vi "Counter 32 Bit (HOST) (SubVI).vi"(5 "Auto RESET":bool=TRUE, 7 "RESET":bool, 8 "Enable":bool, 11 "Max. Count":u32=4294967295) -> (1 "Count End?":bool, 2 "Count Begin?":bool, 3 "Count":u32)   [LabVIEW 2020]
panel:
  # "Counter 32:\n\nCounts when Enable input is TRUE. Count value is 0-indexed."
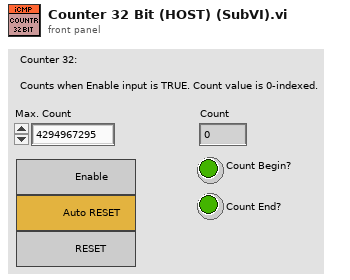
[diagram p1: front panel]
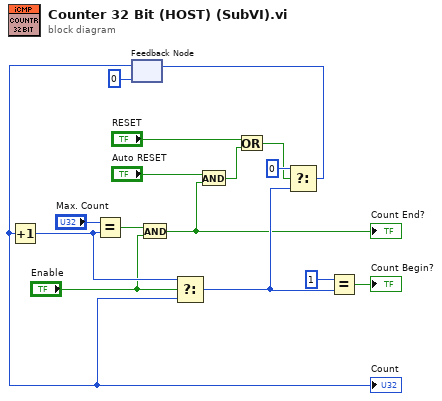
[diagram p0: block diagram]
diagram:
  n1 = feedback #1(u32 0) -> (w16:u32)
  "Count" <- w16
  n2 = Increment(x=w16) -> (x+1=w3:u32)
  n3 = Equal?(x="Max. Count", y=w3) -> (x = y?=w9:bool)
  n4 = And(x=w9, y="Enable") -> (x .and. y?=w2:bool)
  "Count End?" <- w2
  n5 = Select(t=w3, s="Enable", f=w16) -> (s? t:f=w7:u32)
  n6 = And(x="Auto RESET", y=w2) -> (x .and. y?=w5:bool)
  n7 = Or(x="RESET", y=w5) -> (x .or. y?=w4:bool)
  n8 = Select(t=u32 0, s=w4, f=w7) -> (s? t:f=w8:u32)
  n9 = feedback-in #1(w8) -> ()
  n10 = Equal?(x=u32 1, y=w7) -> (x = y?=→"Count Begin?":bool)
